vi "Configure Math Function (Linear).vi"(4 "Math Function Index (1: Math Function 1)":i32(ring)=1 items=["Math Function 1"=1, "Math Function 2"=2, "Math Function 3"=3, "Math Function 4"=4], 8 "error in (no error)":errorcluster, 9 "Linear Offset (0)":dbl, 10 "Linear Gain (1)":dbl=1.0, 11 "VISA resource name":refnum<visa-resource-name>) -> (0 "error out":errorcluster, 3 "VISA resource name out":refnum<visa-resource-name>)   [LabVIEW 2015, in "Agilent 2000 3000 X-Series.lvlib"]
doc: "Configures the linear math function.\n\n<B>Note(s):</B>\nThis VI is applicable for 3000, 3000T, 3000G, 4000, 6000 series."
uses:
  Agilent 2000 3000 X-Series.lvlib
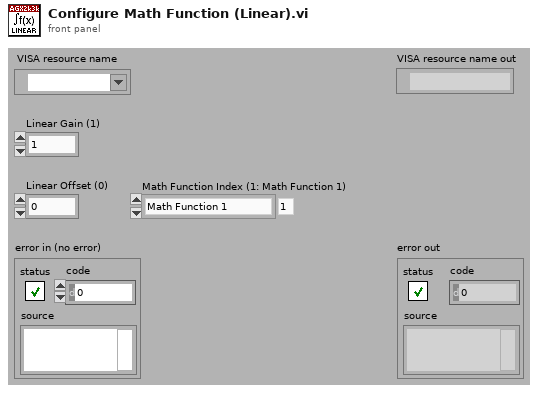
[diagram p1: front panel]
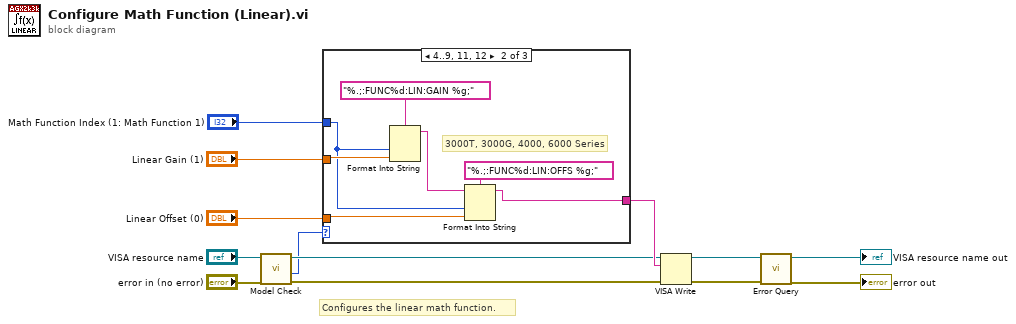
[diagram p0: block diagram]
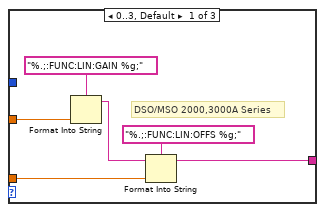
[diagram p2: hidden frame]
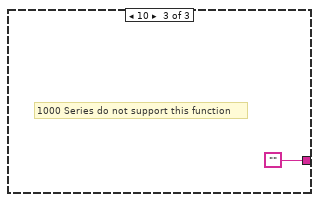
[diagram p3: hidden frame]
diagram:
  # "Configures the linear math function."
  n1 = call "Model Check.vi"("error in (no error)"="error in (no error)", "VISA resource name"="VISA resource name") -> ("error out"=w3:errorcluster, "Model"=w1:i32, "VISA resource name out"=w4:refnum<visa-resource-name>)  [unwired: 7 out]
  n2 = case shown="4..9, 11, 12" w1 {
    tunnel: "Linear Gain (1)" -> [w18 w23 _]
    tunnel: "Linear Offset (0)" -> [w15 w21 _]
    tunnel: [w14 w20 ""] -> w11
    tunnel: "Math Function Index (1: Math Function 1)" -> [_ w22 _]
    frame 0..3, Default {
      # "DSO/MSO 2000,3000A Series"
      n3 = Format Into String(format string="%.;:FUNC:LIN:GAIN %g;", w18) -> (resulting string=w17:string)  [unwired: 2 in, 1 out]
      n4 = Format Into String(format string="%.;:FUNC:LIN:OFFS %g;", initial string=w17, w15) -> (resulting string=w14:string)  [unwired: 1 in, 1 out]
    }
    frame 4..9, 11, 12 {
      # "3000T, 3000G, 4000, 6000 Series"
      n5 = Format Into String(format string="%.;:FUNC%d:LIN:GAIN %g;", w22, w23) -> (resulting string=w25:string)  [unwired: 2 in, 1 out]
      n6 = Format Into String(format string="%.;:FUNC%d:LIN:OFFS %g;", initial string=w25, w22, w21) -> (resulting string=w20:string)  [unwired: 1 in, 1 out]
    }
    frame 10 {
      # "1000 Series do not support this function"
    }
  }
  n7 = VISA Write(VISA resource name=w4, write buffer=w11, error in (no error)=w3) -> (VISA resource name out=w10:refnum<visa-resource-name>, error out=w9:errorcluster)  [unwired: 1 out]
  n8 = call "Error Query.vi"("error in (no error)"=w9, "VISA resource name"=w10) -> ("error out"=→"error out":errorcluster, "VISA resource name out"=→"VISA resource name out":refnum<visa-resource-name>)  [unwired: 8 out]
